vi "FindPropertyNameAndType.vi"(11 "string":string) -> (1 "PropertyFound":bool, 3 "properties":T1)   [LabVIEW 2013, in "CS.lvclass"]
uses:
  CS.lvclass
  baseClass/propertyDef.ctl
  baseClass/types.ctl
  baseClass/baseClass.lvclass
panel:
  out "match + rest of string":string
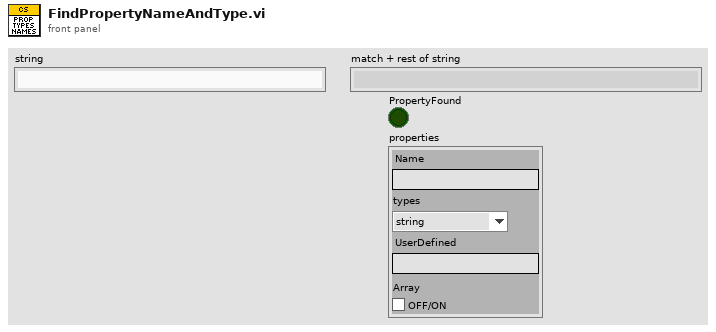
[diagram p1: front panel]
types:
  T1 = typedef "baseClass.lvclass/propertyDef.ctl" = cluster{"Name":string, "types":T2, "UserDefined":string, "Array":bool}
  T2 = typedef "baseClass.lvclass/types.ctl" = enum16{"string", "int", "decimal", "bool", "class", "enum"}
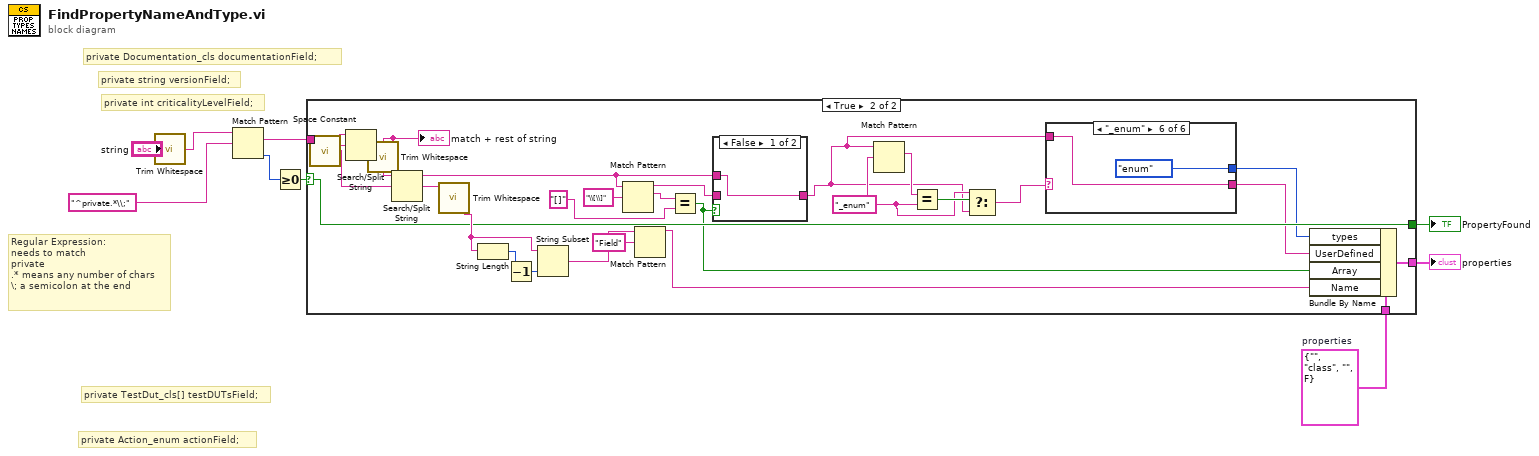
[diagram p0: block diagram]
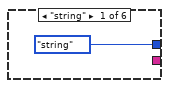
[diagram p3: hidden frame]
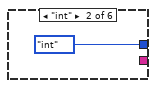
[diagram p4: hidden frame]
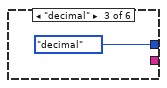
[diagram p5: hidden frame]
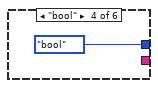
[diagram p6: hidden frame]
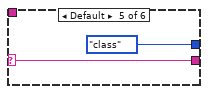
[diagram p7: hidden frame]
diagram:
  w2 = T1 {"Name"="", "types"=enum."class", "UserDefined"="", "Array"=FALSE}  # properties
  # "private Action_enum actionField;"
  # "private TestDut_cls[] testDUTsField;"
  # "Regular Expression:\nneeds to match\nprivate\n.* means any number of chars\n\\; a semicolon at the end"
  # "private int criticalityLevelField;"
  # "private string versionField;"
  # "private Documentation_cls documentationField;"
  n1 = call <vilib>:"Trim Whitespace.vi"("string"="string") -> ("trimmed string"=w3:string)  [unwired: 1 in]
  n2 = Match Pattern(string=w3, regular expression="^private.*\\;") -> (match substring=w6:string, offset past match=w7:i32)  [unwired: 1 in, 2 out]
  n3 = Greater Or Equal To 0?(x=w7) -> (x >= 0?=w5:bool)
  n4 = case shown="True" w5 {
    selector: w5 -> [_ w28]
    tunnel: w6 -> [_ w36]
    tunnel: [_ w28] -> w4
    tunnel: w2 -> [_ w27]
    tunnel: [_ w19] -> w1
    frame False {
    }
    frame True {
      w12 = "_enum" ("regular expression")
      n5 = call <vilib>:"Space Constant.vi"() -> ("String"=w34:string)
      n6 = Search/Split String(string=w36, search string/char (-)=w34) -> (match + rest of string=w35:string)  [unwired: 1 in, 2 out]
      n7 = call <vilib>:"Trim Whitespace.vi"("string"=w35) -> ("trimmed string"=w32:string)  [unwired: 1 in]
      "match + rest of string" <- w32
      n8 = Search/Split String(string=w32, search string/char (-)=w34) -> (substring before match=w23:string, match + rest of string=w33:string)  [unwired: 1 in, 1 out]
      n9 = call <vilib>:"Trim Whitespace.vi"("string"=w33) -> ("trimmed string"=w31:string)  [unwired: 1 in]
      n10 = String Length(string=w31) -> (length=w30:i32)
      n11 = Decrement(x=w30) -> (x-1=w29:i32)
      n12 = String Subset(string=w31, length (rest)=w29) -> (substring=w16:string)  [unwired: 1 in]
      n13 = Match Pattern(string=w23, regular expression="\\[\\]") -> (before substring=w24:string, match substring=w26:string)  [unwired: 1 in, 2 out]
      n14 = Match Pattern(string=w16, regular expression="Field") -> (before substring=w15:string)  [unwired: 1 in, 3 out]
      n15 = Equal?(x=w26, y="[]" ("regular expression")) -> (x = y?=w22:bool)
      n16 = case shown="False" w22 {
        tunnel: w24 -> [_ w46]
        tunnel: [w45 w46] -> w11
        tunnel: w23 -> [w45 _]
        frame False {
        }
        frame True {
        }
      }
      n17 = Match Pattern(string=w11, regular expression=w12) -> (match substring=w14:string)  [unwired: 1 in, 3 out]
      n18 = Equal?(x=w14, y=w12) -> (x = y?=w13:bool)
      n19 = Select(t=w12, s=w13, f=w11) -> (s? t:f=w10:string)
      n20 = case shown="\"_enum\"" w10 {
        selector: w10 -> [_ _ _ _ w42 _]
        tunnel: [_ _ _ _ w42 w43] -> w21
        tunnel: [types."string" ("types") types."int" ("types") types."decimal" ("types") types."bool" ("types") types."class" ("types") types."enum" ("types")] -> w20
        tunnel: w11 -> [_ _ _ _ _ w43]
        frame "string" {
        }
        frame "int" {
        }
        frame "decimal" {
        }
        frame "bool" {
        }
        frame Default {
        }
        frame "_enum" {
        }
      }
      n21 = Bundle By Name(cluster=w27, "types"=w20, "UserDefined"=w21, "Array"=w22, "Name"=w15) -> (w19:T1)
    }
  }
  "PropertyFound" <- w4
  "properties" <- w1
